vi "Calculate conductance ITX.vi"(4 "progress bar?":bool=TRUE, 5 "length":i32=1000, 7 "offset":i32, 9 "index":T2={"N1"=3, "N2"=19, "N3"=4, "N4"=5, "V1"=8, "V2"=8, "V3"=10, "V4"=13, "CURRENT"=4, "Vsg"=1}, 10 "File or Folder Path":path=path "P:/users1/kirkendall/data/SA02835H.20161128/4 - sweep B, Vsg lockin") -> (0 "N Array":T1(array[cluster]), 1 "Comments":string="IGOR\nX// Date: 11/29/2016 8:41 PM\nX// B=-9T to 9T, 100mT steps\nX// Vsg sweep from -200mV to 450mV, 4mV step\nX// Vbg =-2.1V\nX// TC=0.1s\nX// \nX// I+/-: 2/5 25uVac + 360uVdc 13 Hz\nX// V+/-: 3/4\nX// V2+/-: 1/26\nX// appliedB= 89000.000000\n\n\n\n\n\n\n\n\n\n\n\n\n\n\n\n\n\n\n\n\n\n\n\n\n\n\n\n\n\n\n\n\n\n\n\n\n\n\n\n\n\n\n\n\n\n\n\n\n\n\n\n\n\n\n\n\n\n\n\n\n\n\nX \nX Display/R 'time.SA02835H.20161128.000179'\nX AppendToGraph 'Vsg.SA02835H.20161128.000179'\nX AppendToGraph 'T.SA02835H.20161128.000179'\nX AppendToGraph 'B.SA02835H.20161128.000179'\nX AppendToGraph 'X0.SA02835H.20161128.000179'\nX AppendToGraph 'Y0.SA02835H.20161128.000179'\nX AppendToGraph 'X1.SA02835H.20161128.000179'\nX AppendToGraph 'Y1.SA02835H.20161128.000179'\nX AppendToGraph 'X2.SA02835H.20161128.000179'\nX AppendToGraph 'Y2.SA02835H.20161128.000179'\nX AppendToGraph 'X3.SA02835H.20161128.000179'\nX AppendToGraph 'Y3.SA02835H.20161128.000179'\nX AppendToGraph 'X4.SA02835H.20161128.000179'\nX AppendToGraph 'Y4.SA02835H.20161128.000179'\nX AppendToGraph 'X5.SA02835H.20161128.000179'\nX AppendToGraph 'Y5.SA02835H.20161128.000179'\nX AppendToGraph 'X6.SA02835H.20161128.000179'\nX AppendToGraph 'Y6.SA02835H.20161128.000179'\nX AppendToGraph 'X7.SA02835H.20161128.000179'\nX AppendToGraph 'Y7.SA02835H.20161128.000179'\nX AppendToGraph 'X8.SA02835H.20161128.000179'\nX AppendToGraph 'Y8.SA02835H.20161128.000179'\nX AppendToGraph 'X9.SA02835H.20161128.000179'\nX AppendToGraph 'Y9.SA02835H.20161128.000179'\nX AppendToGraph 'Gcalc.SA02835H.20161128.000179'\nX AppendToGraph '25.SA02835H.20161128.000179'\nX AppendToGraph '26.SA02835H.20161128.000179'\nX AppendToGraph '27.SA02835H.20161128.000179'\nX AppendToGraph '28.SA02835H.20161128.000179'\nX AppendToGraph '29.SA02835H.20161128.000179'\nX Label bottom \"x label\"\nX Label left \"y label\"\nX ModifyGraph rgb('time.SA02835H.20161128.000179')=(65280,0,0)\nX ModifyGraph rgb('Vsg.SA02835H.20161128.000179')=(65280,12288,0)\nX ModifyGraph rgb('T.SA02835H.20161128.000179')=(65280,23040,0)\nX ModifyGraph rgb('B.SA02835H.20161128.000179')=(65280,35328,0)\nX ModifyGraph rgb('X0.SA02835H.20161128.000179')=(65280,47616,0)\nX ModifyGraph rgb('Y0.SA02835H.20161128.000179')=(65280,58368,0)\nX ModifyGraph rgb('X1.SA02835H.20161128.000179')=(60416,65280,0)\nX ModifyGraph rgb('Y1.SA02835H.20161128.000179')=(48128,65280,0)\nX ModifyGraph rgb('X2.SA02835H.20161128.000179')=(37376,65280,0)\nX ModifyGraph rgb('Y2.SA02835H.20161128.000179')=(25088,65280,0)\nX ModifyGraph rgb('X3.SA02835H.20161128.000179')=(12800,65280,0)\nX ModifyGraph rgb('Y3.SA02835H.20161128.000179')=(2048,65280,0)\nX ModifyGraph rgb('X4.SA02835H.20161128.000179')=(0,65280,10240)\nX ModifyGraph rgb('Y4.SA02835H.20161128.000179')=(0,65280,22528)\nX ModifyGraph rgb('X5.SA02835H.20161128.000179')=(0,65280,33280)\nX ModifyGraph rgb('Y5.SA02835H.20161128.000179')=(0,65280,45568)\nX ModifyGraph rgb('X6.SA02835H.20161128.000179')=(0,65280,57856)\nX ModifyGraph rgb('Y6.SA02835H.20161128.000179')=(0,62464,65280)\nX ModifyGraph rgb('X7.SA02835H.20161128.000179')=(0,50176,65280)\nX ModifyGraph rgb('Y7.SA02835H.20161128.000179')=(0,37888,65280)\nX ModifyGraph rgb('X8.SA02835H.20161128.000179')=(0,27136,65280)\nX ModifyGraph rgb('Y8.SA02835H.20161128.000179')=(0,14848,65280)\nX ModifyGraph rgb('X9.SA02835H.20161128.000179')=(0,2560,65280)\nX ModifyGraph rgb('Y9.SA02835H.20161128.000179')=(8192,0,65280)\nX ModifyGraph rgb('Gcalc.SA02835H.20161128.000179')=(20480,0,65280)\nX ModifyGraph rgb('25.SA02835H.20161128.000179')=(32768,0,65280)\nX ModifyGraph rgb('26.SA02835H.20161128.000179')=(43520,0,65280)\nX ModifyGraph rgb('27.SA02835H.20161128.000179')=(55808,0,65280)\nX ModifyGraph rgb('28.SA02835H.20161128.000179')=(65280,0,62976)\nX ModifyGraph rgb('29.SA02835H.20161128.000179')=(65280,0,52224)\nX Legend/C/N=text0/J \"\\\\s('time.SA02835H.20161128.000179') time\\r\\\\s('Vsg.SA02835H.20161128.000179') Vsg\\r\\\\s('T.SA02835H.20161128.000179') T\\r\\\\s('B.SA02835H.20161128.000179') B\\r\\\\s('X0.SA02835H.20161128.000179') X0\\r\\\\s('Y0.SA02835H.20161128.000179') Y0\\r\\\\s('X1.SA02835H.20161128.000179') X1\\r\\\\s('Y1.SA02835H.20161128.000179') Y1\\r\\\\s('X2.SA02835H.20161128.000179') X2\\r\\\\s('Y2.SA02835H.20161128.000179') Y2\\r\\\\s('X3.SA02835H.20161128.000179') X3\\r\\\\s('Y3.SA02835H.20161128.000179') Y3\\r\\\\s('X4.SA02835H.20161128.000179') X4\\r\\\\s('Y4.SA02835H.20161128.000179') Y4\\r\\\\s('X5.SA02835H.20161128.000179') X5\\r\\\\s('Y5.SA02835H.20161128.000179') Y5\\r\\\\s('X6.SA02835H.20161128.000179') X6\\r\\\\s('Y6.SA02835H.20161128.000179') Y6\\r\\\\s('X7.SA02835H.20161128.000179') X7\\r\\\\s('Y7.SA02835H.20161128.000179') Y7\\r\\\\s('X8.SA02835H.20161128.000179') X8\\r\\\\s('Y8.SA02835H.20161128.000179') Y8\\r\\\\s('X9.SA02835H.20161128.000179') X9\\r\\\\s('Y9.SA02835H.20161128.000179') Y9\\r\\\\s('Gcalc.SA02835H.20161128.000179') Gcalc\"\nX ModifyGraph mirror(bottom)=1\nX ModifyGraph width=216\nX ModifyGraph height={Aspect,0.6}\nX ModifyGraph Log(bottom)=0\nX ModifyGraph Log(left)=0\nX \n", 2 "A vs D diff":cluster{dbl[], dbl[]}[](graph), 6 "angle phi":dbl[](array[numeric]), 8 "angle theta":dbl[](array[numeric]), 11 "A vs D":cluster{dbl[], dbl[]}[](graph))   [LabVIEW 2016]
uses:
  <vilib>/Utility/miscctls.llb/LVOffsetAndMultiplierTypeDef.ctl
  <vilib>/addons/WireFlow/_WF_ProgressBar.llb/ProgressBar_WireFlow.lvclass
  <userlib>/LevyLab/LV to ITX/LVtoITX.lvclass
  <vilib>/Analysis/NI_AALPro.lvlib
panel:
  out "WF-ProgressBar out":refnum<class "ProgressBar_WireFlow.lvclass">
  in  "Enum":enum16{"Conductance", "Resistance", "Current"}(ring)
  in  "alpha":dbl=0.0150305 format="%#_13g"
  in  "alpha?":bool
  in  "Numeric":dbl=50.0
  in  "dy/dx vs x":bool=TRUE
  in  "single ended?":bool=TRUE
  in  "e^2/h?":bool=TRUE
  in  "log scale?":bool
  in  "calculate Ey":bool=TRUE
  in  "background":enum16{"do nothing", "subtract", "divide"}(ring)
  in  "Background":cluster{dbl[], dbl[]}[](graph)
  in  "A offset":dbl format="%#_6p"
  out "E 2":dbl[][](graph)
  out "counter":i32=89
  out "Path":path=path "P:/users1/kirkendall/data/SA02835H.20161128/4 - sweep B, Vsg lockin/SA02835H.20161128.000179.itx"
  in  "file contains 2D data?":bool
  out "Index, Wavenames":string[][](table)
  out "N":cluster{"N1":dbl, "N2":dbl, "N3":dbl, "N4":dbl}={"N1"=89000.711, "N2"=0.0, "N3"=1.708115564314128e-13, "N4"=7.36783997497257e-13} {"N4" format="%#_6p"; "N3" format="%#_6p"; "N2" format="%#_6p"; "N1" format="%#_20p"}
  in  "Ey":T3={"Offset"=0.0, "Multiplier"=1.0}
  in  "Ex":T3={"Offset"=0.0, "Multiplier"=1.0}
  in  "recolor traces?":bool
  out "C vs D":cluster{dbl[], dbl[]}[](graph)
  out "E":dbl[][](graph)
  in  "B x name":string="Vsg (V)"
  in  "A y name":string="Conductance (S)"
  in  "Ex name":string="Ex name"
  in  "Ez name":string="Ez name"
  in  "D x name":string="Vsg (V)"
  in  "C y name":string="Conductance (S)"
  in  "Ey name":string="Ey name"
  out "time":string[][](table)
  in  "B is time?":bool
  in  "D  is time?":bool
  in  "Generate Folder Index File?":bool
  in  "pattern":string="*.itx"
  in  "Use Folder Index File?":bool
  # "CURRENT/(V1-V2)"
  # "CURRENT/(V3-V4)"
  # "x axis: Vsg\ny axis: single ended?\nT: subtract V1-V2 and V3-V4 and divide by current\nF: plot V1/current"
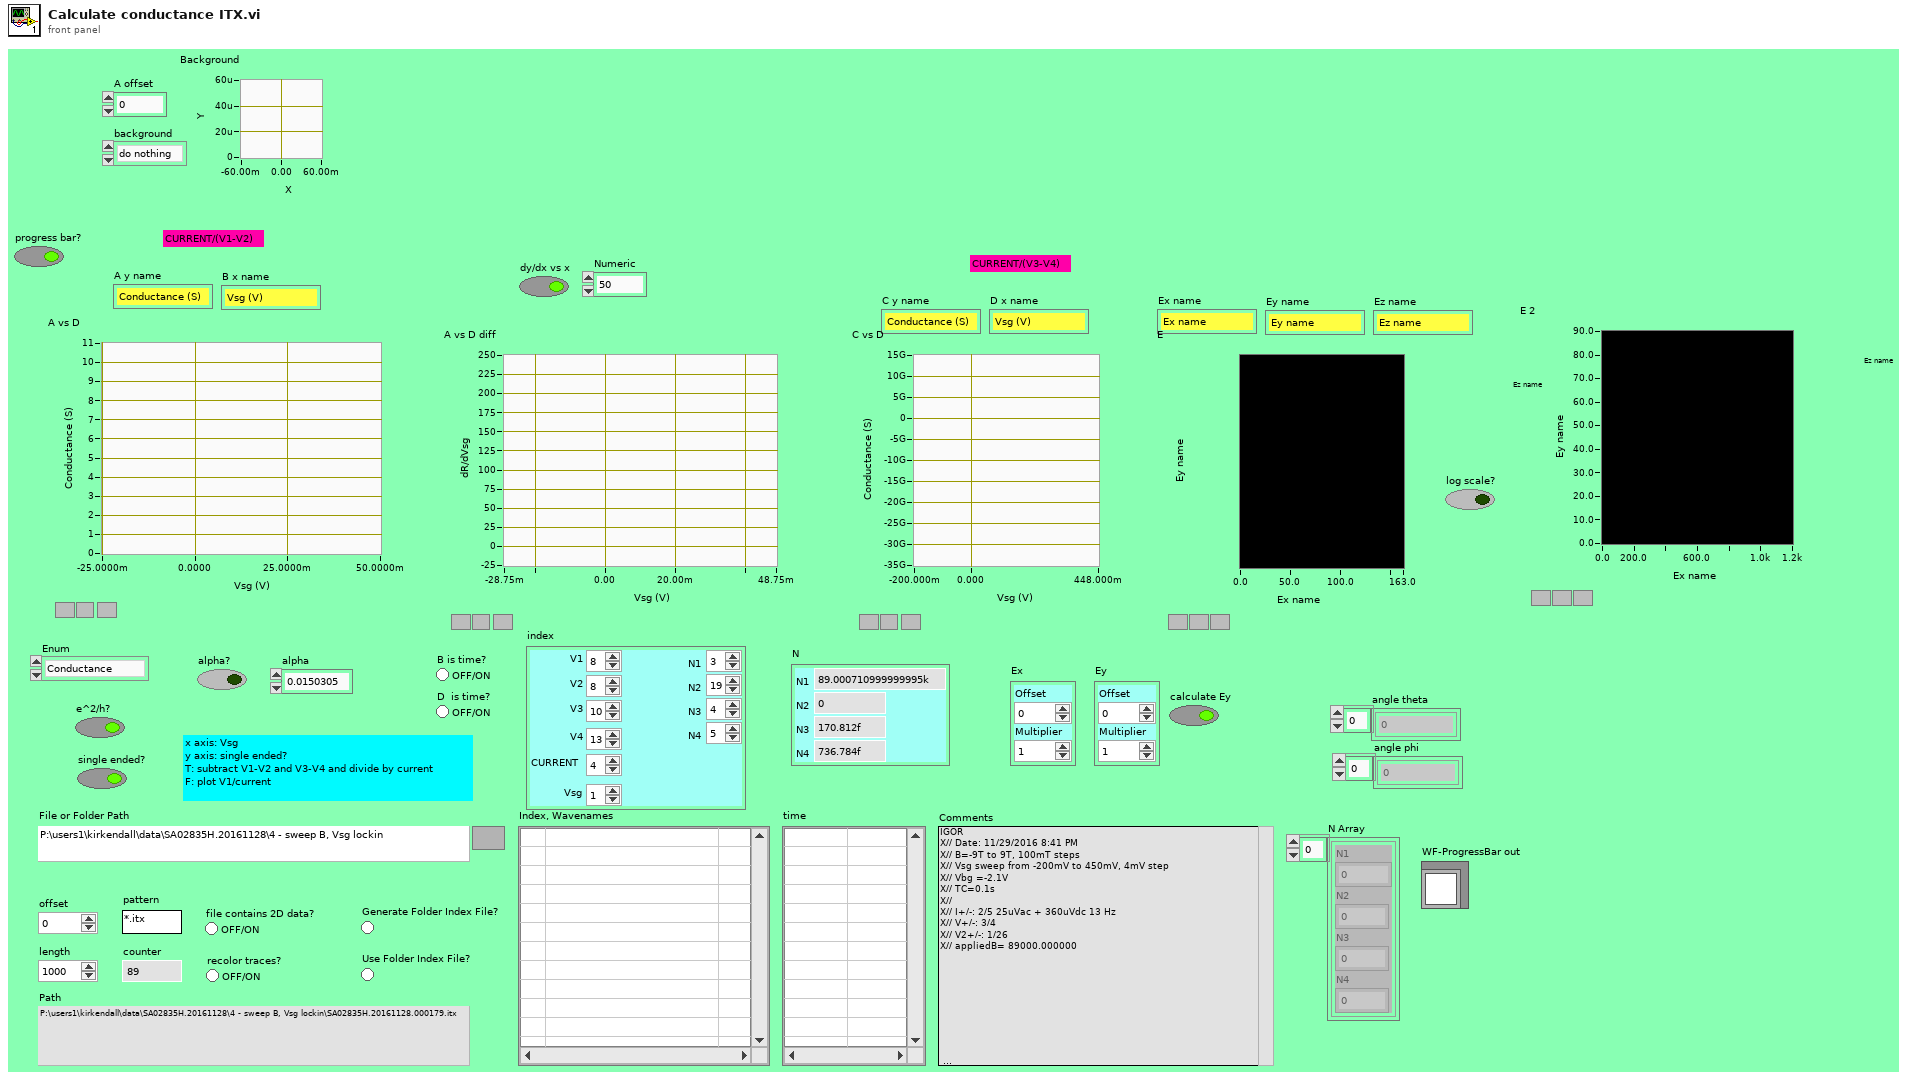
[diagram p1: front panel]
types:
  T1 = cluster{"N1":dbl, "N2":dbl, "N3":dbl, "N4":dbl}[]
  T2 = cluster{"N1":i32, "N2":i32, "N3":i32, "N4":i32, "V1":i32, "V2":i32, "V3":i32, "V4":i32, "CURRENT":i32, "Vsg":i32}
  T3 = typedef "LVOffsetAndMultiplierTypeDef.ctl" = cluster{"Offset":dbl, "Multiplier":dbl}
  T4 = cluster{"Decimated Array":dbl[], "Decimated Array":dbl[]}
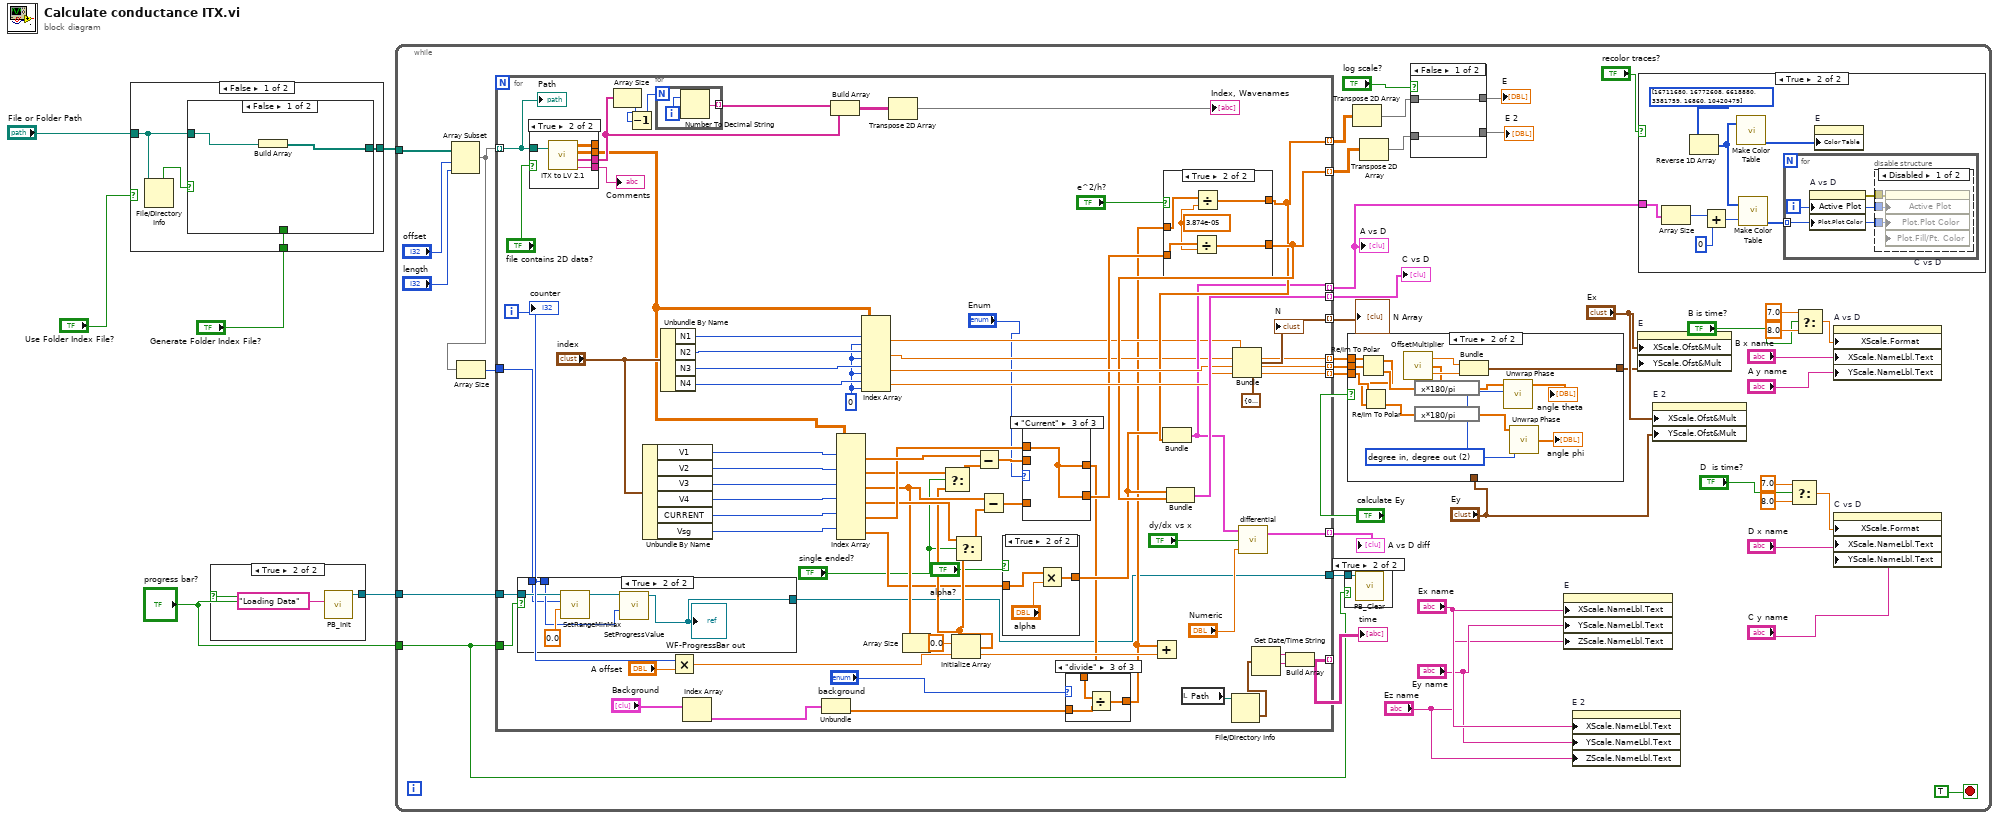
[diagram p0: block diagram]
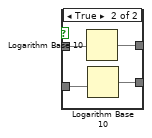
[diagram p4: hidden frame]
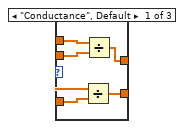
[diagram p11: hidden frame]
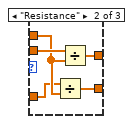
[diagram p12: hidden frame]
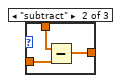
[diagram p14: hidden frame]
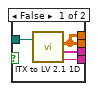
[diagram p15: hidden frame]
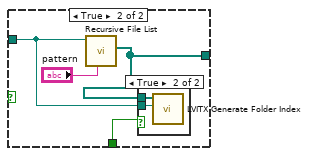
[diagram p16: hidden frame]
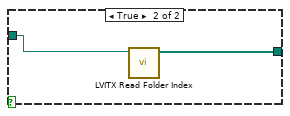
[diagram p18: hidden frame]
diagram:
  n1 = case shown="False" "Use Folder Index File?" {
    tunnel: [w8 w19] -> w4
    tunnel: "File or Folder Path" -> [w10 w20]
    tunnel: "Generate Folder Index File?" -> [w7 _]
    frame False {
      n2 = File/Directory Info(path=w10) -> (directory=w9:bool)  [unwired: 1 in, 6 out]
      n3 = case shown="False" w9 {
        tunnel: [w12 w15] -> w8
        tunnel: w10 -> [w11 w14]
        tunnel: w7 -> [_ w13]
        frame False {
          n4 = Build Array(w11) -> (w12:path[])
        }
        frame True {
          n5 = call <vilib>:"Recursive File List.vi"("pattern"="pattern", "Folder Path"=w14) -> ("All Files in Dir"=w15:path[])  [unwired: 5 in, 4 out]
          n6 = case shown="True" w13 {
            tunnel: w15 -> [_ w18]
            tunnel: w14 -> [_ w17]
            frame False {
            }
            frame True {
              n7 = call <userlib>:"LVITX Generate Folder Index.vi"("File or Folder Path"=w17, "All Files in Dir"=w18) -> ()  [unwired: 10 in]
            }
          }
        }
      }
    }
    frame True {
      n8 = call <userlib>:"LVITX Read Folder Index.vi"("File or Folder Path"=w20) -> ("Array"=w19:path[])  [unwired: 10 in]
    }
  }
  n9 = case shown="True" "progress bar?" {
    tunnel: [_ w22] -> w2
    frame False {
    }
    frame True {
      n10 = call <vilib>:"PB_Init.vi"("title (\"Progress\")"="Loading Data" ("title (\"Progress\")")) -> ("WF-ProgressBar out"=w22:refnum<class "ProgressBar_WireFlow.lvclass">)  [unwired: 9 in, 1 out]
    }
  }
  n11 = while {
    tunnel: w4 -> [w59]
    tunnel: w2 -> [w28]
    tunnel: "progress bar?" -> [w23]
    stop <- TRUE stop-if-true
    n12 = Array Subset(array=w59, index="offset", length="length") -> (w26:path[])
    n13 = Array Size(array=w26) -> (size(s)=w25:i32)
    n14 = for {
      tunnel: w26 -> [w174] mode=indexing
      tunnel: [w174] -> _ mode=indexing
      tunnel: [w157] -> w61 mode=indexing
      tunnel: [w121] -> w49 mode=indexing
      tunnel: [w144] -> w50 mode=indexing
      tunnel: [w131] -> w48 mode=indexing
      tunnel: [w132] -> w47 mode=indexing
      tunnel: [w115] -> w41 mode=indexing
      tunnel: [w136] -> w40 mode=indexing
      tunnel: [w135] -> w39 mode=indexing
      tunnel: [w130] -> w30 mode=indexing
      tunnel: [w118] -> w29 mode=indexing
      tunnel: w28 -> [w107]
      tunnel: w25 -> [w105]
      tunnel: [w104] -> w24
      tunnel: w23 -> [w103]
      i -> [w106]
      w155 = 0 ("disabled index (col)")
      n15 = case shown="True" w103 {
        tunnel: w107 -> [_ w180]
        tunnel: w106 -> [_ w177]
        tunnel: w105 -> [_ w176]
        tunnel: [_ w175] -> w104
        frame False {
        }
        frame True {
          n16 = call-dynamic "SetRangeMinMax.vi"("Min (0)"=0.0, "Max (1)"=w176, "WF-ProgressBar in"=w180) -> ("WF-ProgressBar out"=w178:refnum<class "ProgressBar_WireFlow.lvclass">)  [unwired: 7 in, 1 out]
          n17 = call-dynamic "SetProgressValue.vi"("Value"=w177, "WF-ProgressBar in"=w178) -> ("WF-ProgressBar out"=w175:refnum<class "ProgressBar_WireFlow.lvclass">)  [unwired: 7 in, 2 out]
          "WF-ProgressBar out" <- w175
        }
      }
      n18 = case shown="True" "file contains 2D data?" {
        tunnel: [w215 w218] -> w117
        tunnel: [w213 w219] -> w149
        tunnel: w174 -> [w214 w220]
        tunnel: [w212 w217] -> w167
        tunnel: [w213 w216] -> _
        frame False {
          n19 = call <userlib>:"ITX to LV 2.1 1D.vi"("file (use dialog)"=w214) -> ("array type (2D Dbl)"=w213:dbl[][], "wave names"=w212:string[], "Notes"=w215:string)  [unwired: 2 in]
        }
        frame True {
          n20 = call <userlib>:"ITX to LV 2.1.vi"("file (use dialog)"=w220) -> ("2D array"=w216:dbl[][], "1D arrays"=w219:dbl[][], "wave names"=w217:string[], "Notes"=w218:string)  [unwired: 1 in]
        }
      }
      "Comments" <- w117
      n21 = Array Size(array=w167) -> (size(s)=w170:i32)
      n22 = Decrement(x=w170) -> (x-1=w169:i32)
      n23 = Unbundle By Name("index") -> ("V1"=w154:i32, "V2"=w153:i32, "V3"=w152:i32, "V4"=w151:i32, "CURRENT"=w148:i32, "Vsg"=w143:i32)
      n24 = for {
        N: w169 -> [_]
        tunnel: [w210] -> w172 mode=indexing
        i -> [w211]
        n25 = Number To Decimal String(number=w211) -> (decimal integer string=w210:string)  [unwired: 1 in]
      }
      n26 = Unbundle By Name("index") -> ("N1"=w162:i32, "N2"=w163:i32, "N3"=w164:i32, "N4"=w165:i32)
      n27 = Multiply(x=w106, y="A offset") -> (x*y=w141:dbl)
      n28 = Index Array(array="Background") -> (element=w138:cluster{dbl[], dbl[]})  [unwired: 1 in]
      n29 = Unbundle(w138) -> (w139:dbl[])  [unwired: 1 out]
      n30 = Build Array(w172, w167) -> (w168:string[][])
      n31 = Index Array(array=w149, index (row) #1=w154, index (row) #2=w153, index (row) #3=w152, index (row) #4=w151, index (row) #5=w148, index (row) #6=w143) -> (element #1=w150:dbl[], element #2=w129:dbl[], element #3=w125:dbl[], element #4=w127:dbl[], element #5=w146:dbl[], element #6=w113:dbl[])  [unwired: 6 in]
      n32 = Index Array(array=w149, index (row) #1=w162, index (col) #1=w155, index (row) #2=w163, index (col) #2=w155, index (row) #3=w164, index (col) #3=w155, index (row) #4=w165, index (col) #4=w155) -> (element #1=w116:dbl, element #2=w115:dbl, element #3=w136:dbl, element #4=w135:dbl)
      n33 = Transpose 2D Array(2D array=w168) -> (transposed array=→"Index, Wavenames":string[][])
      n34 = Array Size(array=w125) -> (size(s)=w123:i32)
      n35 = Initialize Array(0.0 ("element"), w123) -> (w122:dbl[])
      n36 = Select(t=w129, s="single ended?", f=w122) -> (s? t:f=w128:dbl[])
      n37 = Select(t=w127, s="single ended?", f=w122) -> (s? t:f=w126:dbl[])
      n38 = Subtract(x=w150, y=w128) -> (x-y=w147:dbl[])
      n39 = Subtract(x=w125, y=w126) -> (x-y=w145:dbl[])
      n40 = case shown="True" "alpha?" {
        tunnel: w113 -> [w181 w184]
        tunnel: [w181 w183] -> w112
        frame False {
        }
        frame True {
          n41 = Multiply(x=w184, y="alpha") -> (x*y=w183:dbl[])
        }
      }
      n42 = case shown="\"Current\"" "Enum" {
        tunnel: w147 -> [w196 w201 _]
        tunnel: w146 -> [w195 w199 w202]
        tunnel: w145 -> [w194 w198 _]
        tunnel: [w193 w197 w202] -> w134
        tunnel: [w192 w200 w202] -> w110
        frame "Conductance", Default {
          n43 = Divide(x=w195, y=w194) -> (x/y=w193:dbl[])
          n44 = Divide(x=w195, y=w196) -> (x/y=w192:dbl[])
        }
        frame "Resistance" {
          n45 = Divide(x=w198, y=w199) -> (x/y=w197:dbl[])
          n46 = Divide(x=w201, y=w199) -> (x/y=w200:dbl[])
        }
        frame "Current" {
        }
      }
      n47 = case shown="\"divide\"" "background" {
        tunnel: w110 -> [w203 w206 w209]
        tunnel: [w203 w205 w207] -> w111
        tunnel: w139 -> [_ w204 w208]
        frame "do nothing", Default {
        }
        frame "subtract" {
          n48 = Subtract(x=w206, y=w204) -> (x-y=w205:dbl[])
        }
        frame "divide" {
          n49 = Divide(x=w209, y=w208) -> (x/y=w207:dbl[])
        }
      }
      n50 = Add(x=w111, y=w141) -> ()  [unwired: 1 out]
      n51 = case shown="True" "e^2/h?" {
        tunnel: w134 -> [w185 w189]
        tunnel: w111 -> [w186 w191]
        tunnel: [w186 w190] -> w131
        tunnel: [w185 w188] -> w132
        frame False {
        }
        frame True {
          w187 = 3.874e-05
          n52 = Divide(x=w189, y=w187) -> (x/y=w188:dbl[])
          n53 = Divide(x=w191, y=w187) -> (x/y=w190:dbl[])
        }
      }
      n54 = Bundle("1D arrays"=w112, "1D arrays"=w131) -> (w121:cluster{"1D arrays":dbl[], "1D arrays":dbl[]})  [unwired: 1 in]
      n55 = Bundle("1D arrays"=w112, "1D arrays"=w132) -> (w144:cluster{"1D arrays":dbl[], "1D arrays":dbl[]})  [unwired: 1 in]
      n56 = local read "Path"() -> (w161:path)
      n57 = File/Directory Info(path=w161) -> (last mod=w160:timestamp)  [unwired: 1 in, 6 out]
      n58 = Bundle(cluster=cluster{"N1":dbl, "N2":dbl, "N3":dbl, "N4":dbl} {"N1"=0.0, "N2"=0.0, "N3"=0.0, "N4"=0.0}, "N1"=w116, "N2"=w115, "N3"=w136, "N4"=w135) -> (w130:cluster{"N1":dbl, "N2":dbl, "N3":dbl, "N4":dbl})
      "N" <- w130
      n59 = call <userlib>:"differential.vi"("Numeric"="Numeric", "dy/dx vs x"="dy/dx vs x", "A vs B 2"=w121) -> ("A vs B 3"=w118:T4)  [unwired: 1 in]
      n60 = Get Date/Time String(seconds (now)=w160) -> (date string=w159:string, time string=w158:string)  [unwired: 2 in]
      n61 = Build Array(w159, w158) -> (w157:string[])
      "counter" <- w106
      "Path" <- w174
    }
    "A vs D" <- w49
    "C vs D" <- w50
    "time" <- w61
    "N Array" <- w30
    "A vs D diff" <- w29
    n62 = case shown="True" w23 {
      tunnel: w24 -> [_ w67]
      frame False {
      }
      frame True {
        n63 = call-dynamic "PB_Clear.vi"("WF-ProgressBar in"=w67) -> ()  [unwired: 9 in, 2 out]
      }
    }
    n64 = case shown="True" "calculate Ey" {
      tunnel: w41 -> [_ w88]
      tunnel: w40 -> [_ w87]
      tunnel: w39 -> [_ w76]
      tunnel: [w74 w83] -> w38
      tunnel: "Ey" -> [w74 _]
      frame False {
      }
      frame True {
        w79 = 2 items=["radian in, radian out", "radian in, degree out", "degree in, degree out", "degree in, radian out"] ("phase unit")
        n65 = Re/Im To Polar(2:w87, 3:w88) -> (0:w86:dbl[], 1:w75:dbl[])
        n66 = Re/Im To Polar(2:w75, 3:w76) -> (0:w77:dbl[])  [unwired: 1 out]
        n67 = expression code="x*180/pi"(w86) -> (w82:dbl[])
        n68 = call <userlib>:"OffsetMultiplier.vi"("Array"=w82) -> ("Offset"=w85:dbl, "Multiplier"=w84:dbl)
        n69 = expression code="x*180/pi"(w77) -> (w80:dbl[])
        n70 = Bundle("Offset"=w85, "Multiplier"=w84) -> (w83:cluster{"Offset":dbl, "Multiplier":dbl})  [unwired: 1 in]
        n71 = call <vilib>:"Unwrap Phase.vi"("phase unit"=w79, "Phase"=w82) -> ("Unwrapped Phase"=→"angle theta":dbl[])  [unwired: 8 in, 1 out]
        n72 = call <vilib>:"Unwrap Phase.vi"("phase unit"=w79, "Phase"=w80) -> ("Unwrapped Phase"=→"angle phi":dbl[])  [unwired: 8 in, 1 out]
      }
    }
    n73 = Transpose 2D Array(2D array=w48) -> (transposed array=w34:dbl[][])
    n74 = Transpose 2D Array(2D array=w47) -> (transposed array=w32:dbl[][])
    n75 = case shown="False" "log scale?" {
      tunnel: w34 -> [w69 w73]
      tunnel: [w69 w72] -> w33
      tunnel: w32 -> [w68 w71]
      tunnel: [w68 w70] -> w31
      frame False {
      }
      frame True {
        n76 = Logarithm Base 10(1:w73) -> (0:w72:dbl[][])
        n77 = Logarithm Base 10(1:w71) -> (0:w70:dbl[][])
      }
    }
    "E" <- w33
    "E 2" <- w31
    n78 = property on="E" class="IntGraph (strict)"("XScale.NameLbl.Text"="Ex name", "YScale.NameLbl.Text"="Ey name", "ZScale.NameLbl.Text"="Ez name") -> ()  [unwired: 2 in, 2 out]
    n79 = property on="E 2" class="IntGraph (strict)"("XScale.NameLbl.Text"="Ex name", "YScale.NameLbl.Text"="Ey name", "ZScale.NameLbl.Text"="Ez name") -> ()  [unwired: 2 in, 2 out]
    n80 = property on="E" class="IntGraph (strict)"("XScale.Ofst&Mult"="Ex", "YScale.Ofst&Mult"=w38) -> ()  [unwired: 2 in, 2 out]
    n81 = case shown="True" "recolor traces?" {
      tunnel: w49 -> [_ w89]
      frame False {
      }
      frame True {
        n82 = Array Size(array=w89) -> (size(s)=w92:i32)
        n83 = Reverse 1D Array(array=u32[] [16711680, 16772608, 6618880, 3381759, 16860, 10420479] ("color scale")) -> (reversed array=w91:u32[])
        n84 = Add(x=w92, y=0 ("x")) -> (x+y=w96:i32)
        n85 = call <userlib>:"Make Color Table.vi"("Array"=w91) -> ("Color Tbl"=w94:u32[])  [unwired: 1 in, 3 out]
        n86 = call <userlib>:"Make Color Table.vi"("Array"=w91, "Size/3"=w96) -> ("Color Tbl"=w93:u32[])  [unwired: 3 out]
        n87 = for {
          tunnel: w93 -> [w97] mode=indexing
          i -> [w98]
          n88 = property on="A vs D" class="XYGraph (strict)"("Active Plot"=w98, "Plot.Plot Color"=w97) -> (error out=w99:errorcluster)  [unwired: 2 in, 1 out]
          n89 = disable-structure shown="Disabled" {
            disable-tunnel: w99 -> [w102 _]
            disable-tunnel: w98 -> [w101 _]
            disable-tunnel: w97 -> [w100 _]
            frame Disabled {
              n90 = property on="C vs D" class="XYGraph (strict)"(error in=w102, "Active Plot"=w101, "Plot.Plot Color"=w100, "Plot.Fill/Pt. Color"=w100) -> ()  [unwired: 1 in, 2 out]
            }
            frame Enabled {
            }
          }
        }
        n91 = property on="E" class="IntGraph (strict)"("Color Table"=w94) -> ()  [unwired: 2 in, 2 out]
      }
    }
    n92 = property on="E 2" class="IntGraph (strict)"("XScale.Ofst&Mult"="Ex", "YScale.Ofst&Mult"="Ey") -> ()  [unwired: 2 in, 2 out]
    n93 = Select(t=7.0, s="D  is time?", f=8.0) -> (s? t:f=w55:dbl)
    n94 = Select(t=7.0, s="B is time?", f=8.0) -> (s? t:f=w56:dbl)
    n95 = property on="A vs D" class="XYGraph (strict)"("XScale.Format"=w56, "XScale.NameLbl.Text"="B x name", "YScale.NameLbl.Text"="A y name") -> ()  [unwired: 2 in, 2 out]
    n96 = property on="C vs D" class="XYGraph (strict)"("XScale.Format"=w55, "XScale.NameLbl.Text"="D x name", "YScale.NameLbl.Text"="C y name") -> ()  [unwired: 2 in, 2 out]
  }
